vi "VariantToProperties.vi"(0 "NHRGridSim in":refnum<class "NHRGridSim.lvclass">, 11 "error in (no error)":errorcluster) -> (4 "NHRGridSim out":refnum<class "NHRGridSim.lvclass">, 6 "Device(s)Settings":T3 {"Modules"."Grid (0: Normal)" items=["Normal", "Grid Emulation"]; "Modules"."Phase (0: All)" items=["All", "A Phase", "B Phase", "C Phase"]; "Modules"."Mode" items=["One 3-Phase AC", "One AC", "One DC", "Three AC", "Three DC", "One 2-Phase AC and One AC", "One 2-Phase AC and One DC", "Two AC", "One AC and One DC", "Two AC and One DC", "One AC and Two DC", "One DC and One AC", "Two DC"]}, 8 "Measurements":T2 {"Phase" items=["All", "A Phase", "B Phase", "C Phase"]}, 10 "MeasName":string, 13 "Measurement Refresh Time (ms)":u32, 14 "Modules":T1 {"Grid (0: Normal)" items=["Normal", "Grid Emulation"]; "Phase (0: All)" items=["All", "A Phase", "B Phase", "C Phase"]; "Mode" items=["One 3-Phase AC", "One AC", "One DC", "Three AC", "Three DC", "One 2-Phase AC and One AC", "One 2-Phase AC and One DC", "Two AC", "One AC and One DC", "Two AC and One DC", "One AC and Two DC", "One DC and One AC", "Two DC"]}, 15 "error out":errorcluster)   [LabVIEW 2018, in "AcPwrPlugins.lvlib" / "NHRGridSim.lvclass"]
uses:
  NHRGridSim.lvclass
  C:/Users/ico/Documents/Projects/NistPluggableModules/AcPwr/AcPwrPlugins/AcPwrBaseClass/AcPwrBase.lvclass
  TypeDefs/DeviceSettings.ctl
  TypeDefs/Modules.ctl
  Measurements.ctl
  AcPwrBaseClass/AcPwrBase.lvclass/AcPwrBase.ctl
  AcPwrBaseClass/Accessors/Read BaseConfig.vi
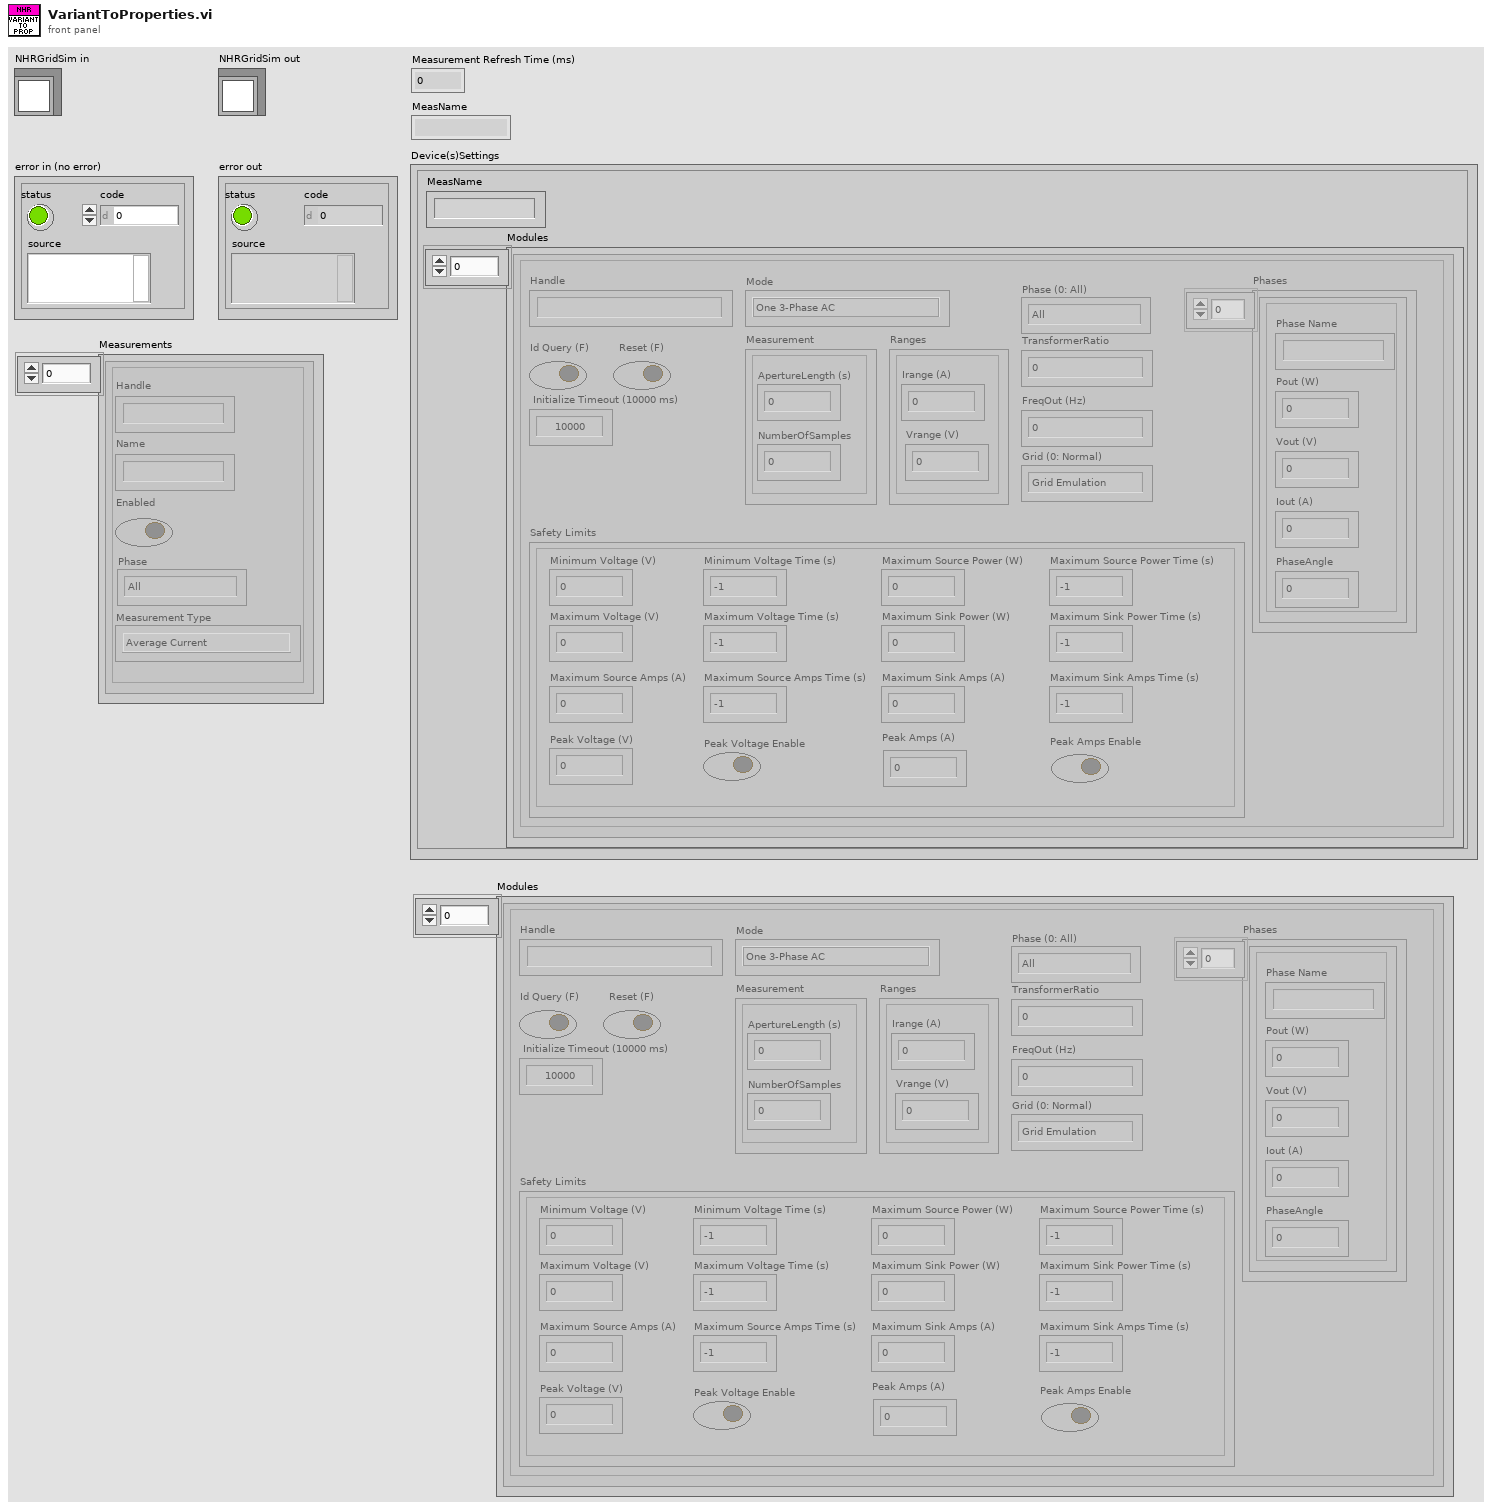
[diagram p1: front panel]
types:
  T1 = typedef "AcPwrPlugins.lvlib/NHRGridSim.lvclass/Modules.ctl" = cluster{"Measurement":cluster{"ApertureLength (s)":dbl, "NumberOfSamples":u32}, "Ranges":cluster{"Irange (A)":dbl, "Vrange (V)":dbl}, "Mode":u8, "TransformerRatio":dbl, "Handle":string, "FreqOut (Hz)":dbl, "Connected":bool, "btnIdQuery":bool, "btnReset":bool, "Initialize Timeout (10000 ms)":u32, "Phase (0: All)":i32, "Safety Limits":cluster{"Minimum Voltage (V)":dbl, "Minimum Voltage Time (s)":dbl, "Maximum Voltage (V)":dbl, "Maximum Voltage Time (s)":dbl, "Maximum Source Amps (A)":dbl, "Maximum Source Amps Time (s)":dbl, "Maximum Sink Amps (A)":dbl, "Maximum Sink Amps Time (s)":dbl, "Maximum Source Power (W)":dbl, "Maximum Source Power Time (s)":dbl, "Maximum Sink Power (W)":dbl, "Maximum Sink Power Time (s)":dbl, "Peak Voltage (V)":dbl, "Peak Voltage Enable":bool, "Peak Amps (A)":dbl, "Peak Amps Enable":bool}, "Grid (0: Normal)":i32, "Phases":cluster{"Pout (W)":dbl, "Iout (A)":dbl, "PhaseAngle":dbl, "Vout (V)":dbl, "Phase Name":string}[]}[]
  T2 = typedef "AcPwrPlugins.lvlib/NHRGridSim.lvclass/Measurements.ctl" = cluster{"Handle":string, "Name":string, "Enabled ":bool, "Measurement Value":dbl, "Measurement Type ":enum16{"Average Current", "Max Current", "Min Current", "Average Voltage", "Max Voltage", "Min Voltage", "Average True Power", "Max True Power", "Min True Power", "Average Apparent Power", "Max Apparent Power", "Min Apparent Power", "Power Factor", "Crest Factor"}, "Phase ":i32}[]
  T3 = typedef "AcPwrPlugins.lvlib/NHRGridSim.lvclass/DeviceSettings.ctl" = cluster{"MeasName":string, "Modules":T1}
  T4 = typedef "AcPwrPlugins.lvlib/AcPwrBase.lvclass/BaseConfig.ctl" = cluster{"Frequency":dbl, "FrequencyRange":dbl[], "Phases":T5[], "Name":string, "PluginConfigVariant":variant, "PluginMeasVariant":variant}
  T5 = typedef "AcPwrPlugins.lvlib/AcPwrBase.lvclass/Phase.ctl" = cluster{"Name":string, "Enabled":bool, "VoltageLevel":dbl, "Handle":string, "VoltageRange":dbl[], "Connected":bool, "CurrentLimit":dbl, "Waveform":string}
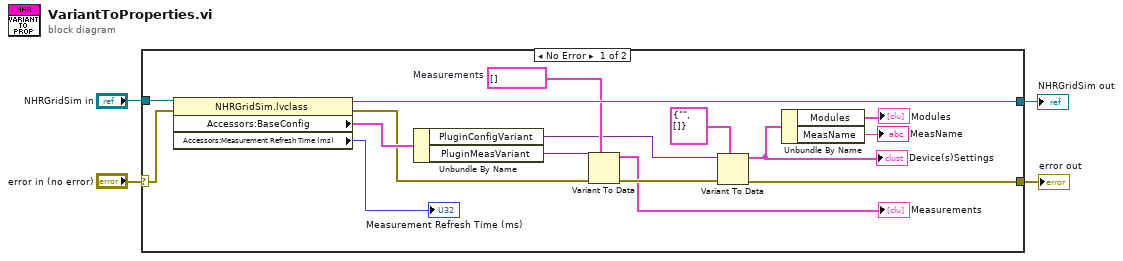
[diagram p0: block diagram]
diagram:
  n1 = case shown="No Error" "error in (no error)" {
    selector: "error in (no error)" -> [w18 w22]
    tunnel: [w20 w22] -> w1
    tunnel: "NHRGridSim in" -> [w19 w21]
    tunnel: [w17 w21] -> w2
    frame No Error {
      w10 = T2 []  # Measurements
      n2 = property class="NHRGridSim.lvclass"(reference=w19, error in=w18) -> (reference out=w17:refnum<class "NHRGridSim.lvclass">, error out=w13:errorcluster, "Accessors:BaseConfig"=w16:T4, "Accessors:Measurement Refresh Time (ms)"=→"Measurement Refresh Time (ms)":u32)
      n3 = Unbundle By Name(w16) -> ("PluginConfigVariant"=w8:variant, "PluginMeasVariant"=w11:variant)
      n4 = Variant To Data(error in=w13, type=w10, Variant=w11) -> (data=→"Measurements":T2, error out=w12:errorcluster)
      n5 = Variant To Data(error in=w12, type=T3 {"MeasName"="", "Modules"=[]} ("Device(s)Settings"), Variant=w8) -> (data=w15:T3, error out=w20:errorcluster)
      "Device(s)Settings" <- w15
      n6 = Unbundle By Name(w15) -> ("Modules"=→"Modules":T1, "MeasName"=→"MeasName":string)
    }
    frame Error {
    }
  }
  "error out" <- w1
  "NHRGridSim out" <- w2
